vi "Load Settings.vi"(4 "error in (not an error)":errorcluster, 7 "config file":path) -> (0 "error out":errorcluster, 1 "channels":T2[](array[typedef]) {"input config" items=["no change", "differential", "ref. single-ended", "non-ref. single-ended", "4-wire"]; "coupling" items=["no change", "DC", "AC", "GND", "internal ref."]; "engineering units" items=["custom...", "V", "Pa", "g", "m/s^2", "m/s", "m", "in/s^2", "in/s", "in"]; "sensor sensitivity (mV/EU)" format="%.2f"; "range(+_)" format="%.2f"}, 2 "parameters":T1 {"sample rate" format="%.2f"}, 3 "config file out":path)   [LabVIEW 2017]
uses:
  <vilib>/addons/Sound and Vibration/Order Analysis/Misc/OAT Channel Setting.ctl
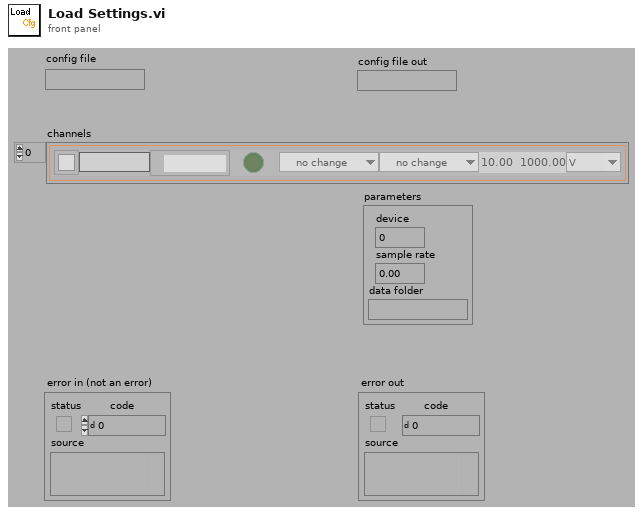
[diagram p1: front panel]
types:
  T1 = cluster{"device":i16, "sample rate":sgl, "data folder":path}
  T2 = typedef "OAT Channel Setting.ctl" = cluster{"color":u32, "name":string, "channel":tag, "coupling":u16, "input config":u16, "range(+_)":sgl, "sensor sensitivity (mV/EU)":dbl, "engineering units":u16, "excitation":bool}
  T3 = cluster{"Device":i16, "Sample rate":sgl, "Data folder":path}
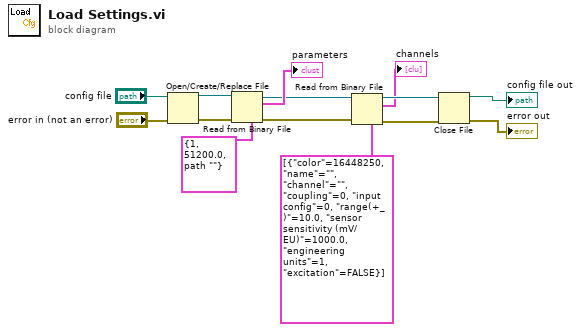
[diagram p0: block diagram]
diagram:
  n1 = Open/Create/Replace File(file path (use dialog)="config file", error in="error in (not an error)") -> (refnum out=w1:refnum<file>, error out=w10:errorcluster)  [unwired: 4 in, 1 out]
  n2 = Read from Binary File(5:T3 {"Device"=1, "Sample rate"=51200.0, "Data folder"=path ""}, 8:w10, 11:w1) -> (0:w8:errorcluster, 2:→"parameters":T3, 3:w9:refnum<file>)  [unwired: 3 in, 1 out]
  n3 = Read from Binary File(5:T2[] [{"color"=16448250, "name"="", "channel"="", "coupling"=0, "input config"=0, "range(+_)"=10.0, "sensor sensitivity (mV/EU)"=1000.0, "engineering units"=1, "excitation"=FALSE}] ("Channels"), 8:w8, 11:w9) -> (0:w6:errorcluster, 2:→"channels":T2[], 3:w7:refnum<file>)  [unwired: 3 in, 1 out]
  n4 = Close File(refnum=w7, error in=w6) -> (path=→"config file out":path, error out=→"error out":errorcluster)
